vi "Get Attribute BOOL.vi"(8 "error in":errorcluster, 10 "Attribute":string, 11 "IConfigure in":refnum<class "IConfigure.lvclass">) -> (0 "error out":errorcluster, 2 "Value":bool, 3 "IConfigure out":refnum<class "IConfigure.lvclass">)   [LabVIEW 2024, in "IConfigure.lvclass"]
uses:
  IConfigure.lvclass
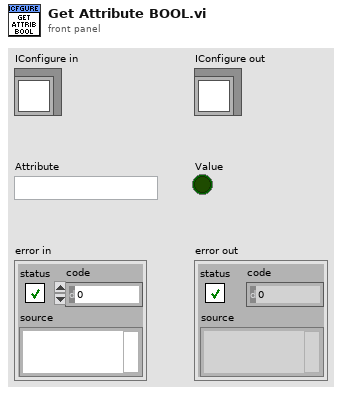
[diagram p1: front panel]
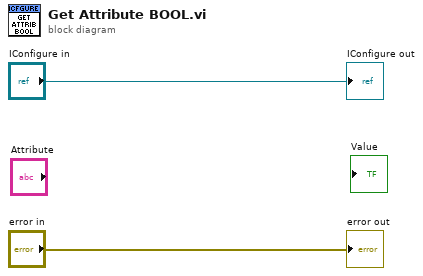
[diagram p0: block diagram]
diagram:
  "error out" <- "error in"
  "IConfigure out" <- "IConfigure in"
